vi "update.vi"(8 "error in (no error)":errorcluster, 10 "Model in":refnum<class "Model.lvclass">, 11 "StandbyState in":refnum<class "StandbyState.lvclass">) -> (0 "error out":errorcluster, 2 "Model out":refnum<class "Model.lvclass">, 3 "StandbyState out":refnum<class "StandbyState.lvclass">)   [LabVIEW 2016, in "StandbyState.lvclass"]
uses:
  StandbyState.lvclass
  Model/Model.lvclass
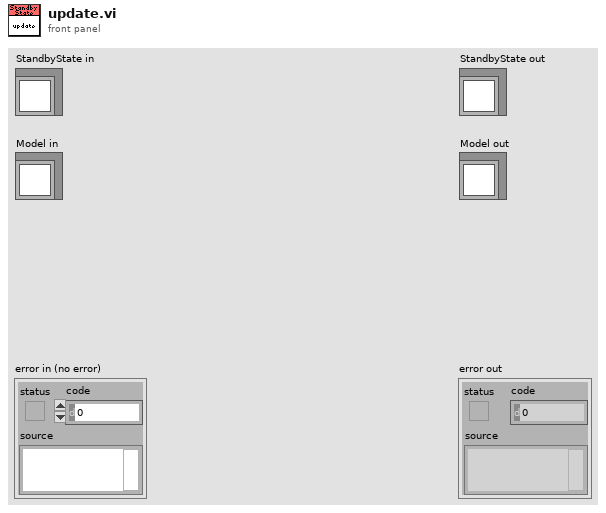
[diagram p1: front panel]
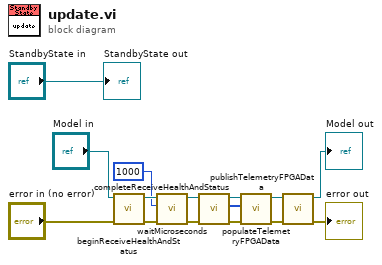
[diagram p0: block diagram]
diagram:
  n1 = call "beginReceiveHealthAndStatus.vi"("error in (no error)"="error in (no error)", "Model in"="Model in") -> ("error out"=w4:errorcluster, "Model out"=w10:refnum<class "Model.lvclass">)  [unwired: 8 in]
  n2 = call "waitMicroseconds.vi"("error in (no error)"=w4, "Time (us)"=u32 1000, "Model in"=w10) -> ("error out"=w3:errorcluster, "Model out"=w8:refnum<class "Model.lvclass">)  [unwired: 7 in]
  n3 = call "completeReceiveHealthAndStatus.vi"("error in (no error)"=w3, "Model in"=w8) -> ("error out"=w14:errorcluster, "Data"=w15:u32[], "Model out"=w13:refnum<class "Model.lvclass">)  [unwired: 7 in]
  n4 = call "populateTelemetryFPGAData.vi"("error in (no error)"=w14, "Data"=w15, "Model in"=w13) -> ("error out"=w2:errorcluster, "Model out"=w7:refnum<class "Model.lvclass">)  [unwired: 7 in]
  n5 = call "publishTelemetryFPGAData.vi"("error in (no error)"=w2, "Model in"=w7) -> ("error out"=→"error out":errorcluster, "Model out"=→"Model out":refnum<class "Model.lvclass">)  [unwired: 8 in]
  "StandbyState out" <- "StandbyState in"
